vi "read_wav_from_txt.vi"(11 "名称或相对路径":string) -> (0 "error out":errorcluster caption="错误输出", 2 "wav":dbl[](array[numeric]) caption="第一行")   [LabVIEW 2018]
uses:
  <vilib>/Utility/file.llb/Read Delimited Spreadsheet (DBL).vi
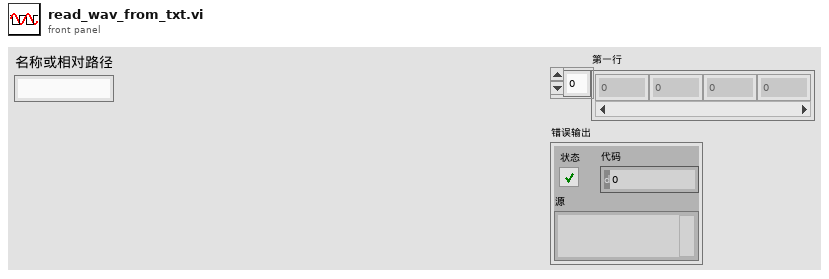
[diagram p1: front panel]
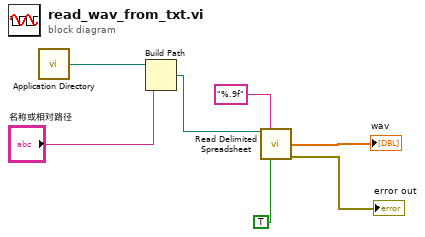
[diagram p0: block diagram]
diagram:
  n1 = call <vilib>:"Application Directory.vi"() -> ("Application Directory"=w1:path)
  n2 = Build Path(base path=w1, name or relative path="名称或相对路径") -> (appended path=w2:path)
  n3 = call-poly <vilib>:"Read Delimited Spreadsheet.vi"("file path (dialog if empty)"=w2, "format (%.3f)"="%.9f", "transpose? (F)"=TRUE) -> ("first row"=→"wav":dbl[], "error out"=→"error out":errorcluster)  [unwired: 7 in, 4 out]
